vi "Initialize.vi"() -> (0 "Error Out":errorcluster, 3 "Revert Worker Config":T1={"Job Queue"=refnum, "Job Done Queue"=refnum, "Source File Name"="", "Output Path"="", "Source Directory"=path "", "Unzip Directory"=path "", "Backsave Directory"=path "", "Output Directory"=path "", "LabVIEW Version"=enum."13.0"})   [LabVIEW 2013, in "LVH-Revert.lvlib"]
uses:
  <vilib>/LabVIEW Hacker/Revert/LVH-Revert.lvlib
  <vilib>/LabVIEW Hacker/Revert/Private/Revert Worker Config.ctl
  <vilib>/National Instruments/LabVIEW 2012 AWS Toolkit/SQS/VI Source/AWS SQS Class/AWS_SQS.lvclass
  <vilib>/National Instruments/LabVIEW 2012 AWS Toolkit/AWS Core Lib/VI Source/Canonicals/AWS_Core Canonical Credentials/Canonical Credentials.lvclass
  <vilib>/National Instruments/LabVIEW 2012 AWS Toolkit/AWS Core Lib/VI Source/Canonicals/AWS_Core Canonical Required Parameters/Canonical Required Parameters.lvclass
  <vilib>/National Instruments/LabVIEW 2012 AWS Toolkit/SQS/VI Source/Canonicals/Canonical CreateQueue/Canonical CreateQueue.lvclass
  <vilib>/National Instruments/LabVIEW 2012 AWS Toolkit/SQS/VI Source/Canonicals/Canonical ListQueues/Canonical ListQueues.lvclass
  <vilib>/National Instruments/LabVIEW 2012 AWS Toolkit/SQS/VI Source/Canonicals/Canonical AddPermission/Canonical AddPermission.lvclass
  <vilib>/National Instruments/LabVIEW 2012 AWS Toolkit/SQS/VI Source/Canonicals/Canonical ChangeMessageVisibility/Canonical ChangeMessageVisibility.lvclass
  <vilib>/National Instruments/LabVIEW 2012 AWS Toolkit/SQS/VI Source/Canonicals/Canonical ChangeMessageVisibilityBatch/Canonical ChangeMessageVisibilityBatch.lvclass
  <vilib>/National Instruments/LabVIEW 2012 AWS Toolkit/SQS/VI Source/Canonicals/Canonical DeleteMessage/Canonical DeleteMessage.lvclass
  <vilib>/National Instruments/LabVIEW 2012 AWS Toolkit/SQS/VI Source/Canonicals/Canonical DeleteMessageBatch/Canonical DeleteMessageBatch.lvclass
  <vilib>/National Instruments/LabVIEW 2012 AWS Toolkit/SQS/VI Source/Canonicals/Canonical GetQueueAttributes/Canonical GetQueueAttributes.lvclass
  <vilib>/National Instruments/LabVIEW 2012 AWS Toolkit/SQS/VI Source/Canonicals/Canonical GetQueueUrl/Canonical GetQueueUrl.lvclass
  <vilib>/National Instruments/LabVIEW 2012 AWS Toolkit/SQS/VI Source/Canonicals/Canonical ReceiveMessage/Canonical ReceiveMessage.lvclass
  <vilib>/National Instruments/LabVIEW 2012 AWS Toolkit/SQS/VI Source/Canonicals/Canonical RemovePermission/Canonical RemovePermission.lvclass
  <vilib>/National Instruments/LabVIEW 2012 AWS Toolkit/SQS/VI Source/Canonicals/Canonical SendMessage/Canonical SendMessage.lvclass
  <vilib>/National Instruments/LabVIEW 2012 AWS Toolkit/SQS/VI Source/Canonicals/Canonical SendMessageBatch/Canonical SendMessageBatch.lvclass
  <vilib>/National Instruments/LabVIEW 2012 AWS Toolkit/SQS/VI Source/Canonicals/Canonical SetQueueAttributes/Canonical SetQueueAttributes.lvclass
  <vilib>/LabVIEW Hacker/LVH-Toolbox/Common/Private/Type Defs/LabVIEW Version.ctl
  <vilib>/National Instruments/LabVIEW 2012 AWS Toolkit/AWS Core Lib/VI Source/Typedefs/AWS_AWS Credentials.ctl
  <vilib>/National Instruments/LabVIEW 2012 AWS Toolkit/SQS/VI Source/Public Typedefs/AWS_SQS Queue Name and Account Number.ctl
  <vilib>/Utility/config.llb/Read Key (String).vi
  <vilib>/Utility/config.llb/Read Key (Path).vi
  <vilib>/Utility/config.llb/NI_LVConfig.lvlib
  <vilib>/National Instruments/LabVIEW 2012 AWS Toolkit/AWS Core Lib/VI Source/AWS_Core.lvlib
  <vilib>/National Instruments/LabVIEW 2012 AWS Toolkit/SQS/VI Source/AWS_SQS.lvlib
  <vilib>/National Instruments/LabVIEW Interface for Amazon S3/LV Interface for Amazon S3.lvlib
  <vilib>/LabVIEW Hacker/LVH-Toolbox/Common/LVH-Common.lvlib
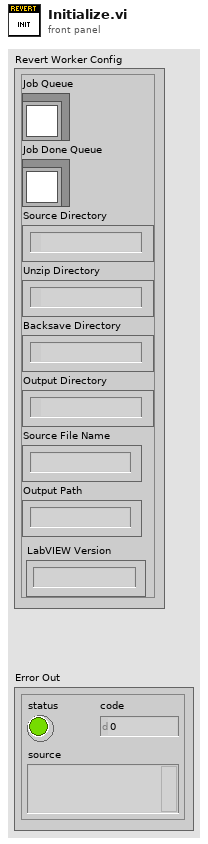
[diagram p1: front panel]
types:
  T1 = typedef "LVH-Revert.lvlib/Revert Worker Config.ctl" = cluster{"Job Queue":refnum<class "AWS_SQS.lvclass">, "Job Done Queue":refnum<class "AWS_SQS.lvclass">, "Source File Name":string, "Output Path":string, "Source Directory":path, "Unzip Directory":path, "Backsave Directory":path, "Output Directory":path, "LabVIEW Version":T2}
  T2 = typedef "LVH-Toolbox.lvlib/LVH-Common.lvlib/LabVIEW Version.ctl" = enum16{"8.0", "8.2", "8.6", "9.0", "10.0", "11.0", "12.0", "13.0"}
  T3 = typedef "AWS_SQS.lvlib/AWS_SQS Queue Name and Account Number.ctl" = cluster{"QueueName":string, "Account Number":string}
  T4 = typedef "AWS_Core.lvlib/AWS_AWS Credentials.ctl" = cluster{"AWSAccessKeyId":string, "Secret Key":string}
  T5 = typedef "NI_LVConfig.lvlib/Config Data RefNum.ctl" = refnum<k1>
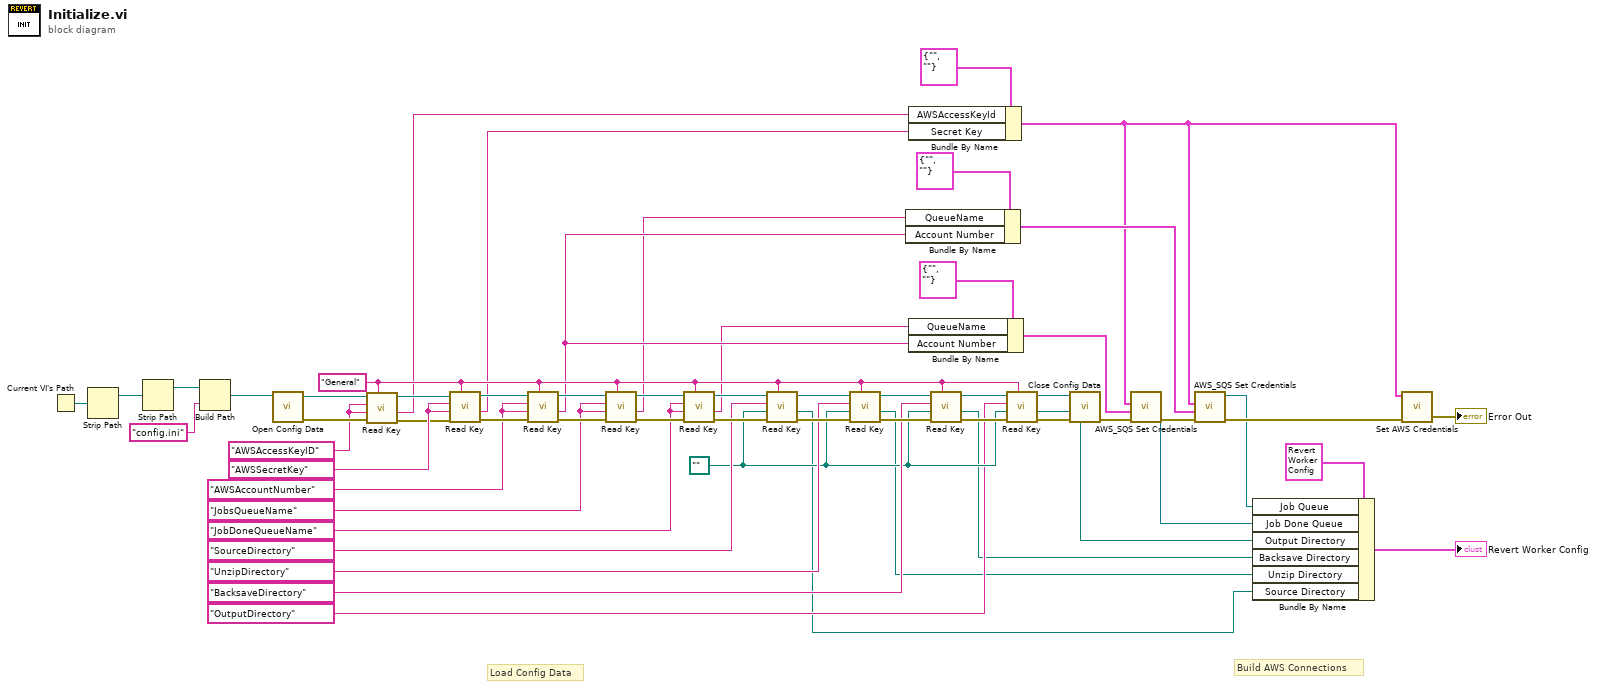
[diagram p0: block diagram]
diagram:
  w43 = path "" ("Unzip Directory")
  w47 = "JobDoneQueueName"
  w48 = "JobsQueueName"
  w49 = "AWSAccountNumber"
  w50 = "AWSSecretKey"
  w51 = "AWSAccessKeyID"
  w32 = "General" ("section")
  # "Build AWS Connections"
  # "Load Config Data"
  n1 = Current VI's Path() -> (path=w30:path)
  n2 = Strip Path(path=w30) -> (stripped path=w29:path)  [unwired: 1 out]
  n3 = Strip Path(path=w29) -> (stripped path=w28:path)  [unwired: 1 out]
  n4 = Build Path(base path=w28, name or relative path="config.ini") -> (appended path=w26:path)
  n5 = call <vilib>:"Open Config Data.vi"("configuration file path"=w26) -> ("error out"=w59:errorcluster, "refnum"=w34:T5)  [unwired: 8 in, 1 out]
  n6 = call-poly <vilib>:"Read Key.vi"("section"=w32, "error in (no error)"=w59, "default value"=w51, "key"=w51, "refnum"=w34) -> ("error out"=w35:errorcluster, "value"=w22:string, "refnum out"=w33:T5)  [unwired: 3 in, 1 out]
  n7 = call-poly <vilib>:"Read Key.vi"("section"=w32, "error in (no error)"=w35, "default value"=w50, "key"=w50, "refnum"=w33) -> ("error out"=w58:errorcluster, "value"=w21:string, "refnum out"=w42:T5)  [unwired: 3 in, 1 out]
  n8 = call-poly <vilib>:"Read Key.vi"("section"=w32, "error in (no error)"=w58, "default value"=w49, "key"=w49, "refnum"=w42) -> ("error out"=w57:errorcluster, "value"=w18:string, "refnum out"=w41:T5)  [unwired: 3 in, 1 out]
  n9 = call-poly <vilib>:"Read Key.vi"("section"=w32, "error in (no error)"=w57, "default value"=w48, "key"=w48, "refnum"=w41) -> ("error out"=w56:errorcluster, "value"=w17:string, "refnum out"=w40:T5)  [unwired: 3 in, 1 out]
  n10 = call-poly <vilib>:"Read Key.vi"("section"=w32, "error in (no error)"=w56, "default value"=w47, "key"=w47, "refnum"=w40) -> ("error out"=w55:errorcluster, "value"=w16:string, "refnum out"=w39:T5)  [unwired: 3 in, 1 out]
  n11 = call-poly <vilib>:"Read Key.vi"("section"=w32, "error in (no error)"=w55, "default value"=w43, "key"="SourceDirectory", "refnum"=w39) -> ("error out"=w54:errorcluster, "value"=w7:path, "refnum out"=w38:T5)  [unwired: 3 in, 1 out]
  n12 = call-poly <vilib>:"Read Key.vi"("section"=w32, "error in (no error)"=w54, "default value"=w43, "key"="UnzipDirectory", "refnum"=w38) -> ("error out"=w53:errorcluster, "value"=w8:path, "refnum out"=w37:T5)  [unwired: 3 in, 1 out]
  n13 = Bundle By Name(cluster=T3 {"QueueName"="", "Account Number"=""} ("Queue Name and Account Number"), "QueueName"=w17, "Account Number"=w18) -> (w15:T3)
  n14 = Bundle By Name(cluster=T4 {"AWSAccessKeyId"="", "Secret Key"=""} ("AWS Credentials"), "AWSAccessKeyId"=w22, "Secret Key"=w21) -> (w13:T4)
  n15 = Bundle By Name(cluster=T3 {"QueueName"="", "Account Number"=""} ("Queue Name and Account Number"), "QueueName"=w16, "Account Number"=w18) -> (w1:T3)
  n16 = call-poly <vilib>:"Read Key.vi"("section"=w32, "error in (no error)"=w53, "default value"=w43, "key"="BacksaveDirectory", "refnum"=w37) -> ("error out"=w52:errorcluster, "value"=w9:path, "refnum out"=w36:T5)  [unwired: 3 in, 1 out]
  n17 = call-poly <vilib>:"Read Key.vi"("section"=w32, "error in (no error)"=w52, "default value"=w43, "key"="OutputDirectory", "refnum"=w36) -> ("error out"=w5:errorcluster, "value"=w10:path, "refnum out"=w3:T5)  [unwired: 3 in, 1 out]
  n18 = call <vilib>:"Close Config Data.vi"("error in (no error)"=w5, "refnum"=w3) -> ("error out"=w4:errorcluster)  [unwired: 8 in, 1 out]
  n19 = call <vilib>:"AWS_SQS Set Credentials.vi"("error in (no error)"=w4, "Queue Name and Account Number"=w1, "AWS Credentials"=w13) -> ("error out"=w25:errorcluster, "AWS_SQS out"=w11:refnum<class "AWS_SQS.lvclass">)  [unwired: 7 in]
  n20 = call <vilib>:"AWS_SQS Set Credentials.vi"("error in (no error)"=w25, "Queue Name and Account Number"=w15, "AWS Credentials"=w13) -> ("error out"=w14:errorcluster, "AWS_SQS out"=w12:refnum<class "AWS_SQS.lvclass">)  [unwired: 7 in]
  n21 = Bundle By Name(cluster=T1 {"Job Queue"=refnum, "Job Done Queue"=refnum, "Source File Name"="", "Output Path"="", "Source Directory"=path "", "Unzip Directory"=path "", "Backsave Directory"=path "", "Output Directory"=path "", "LabVIEW Version"=enum."8.0"} ("Revert Worker Config"), "Job Queue"=w12, "Job Done Queue"=w11, "Output Directory"=w10, "Backsave Directory"=w9, "Unzip Directory"=w8, "Source Directory"=w7) -> (→"Revert Worker Config":T1)
  n22 = call <vilib>:"Set AWS Credentials.vi"("error in (no error)"=w14, "AWS Credentials in"=w13) -> ("error out"=→"Error Out":errorcluster)  [unwired: 9 in]
